vi "Pre-Build Failure Tests.vi"(8 "error in (no error)":errorcluster, 11 "Pre-Build Properties":T1) -> (0 "error out":errorcluster, 3 "Pre-Build Properties dup":T1)   [LabVIEW 2013]
uses:
  pre-build properties -- cluster.ctl
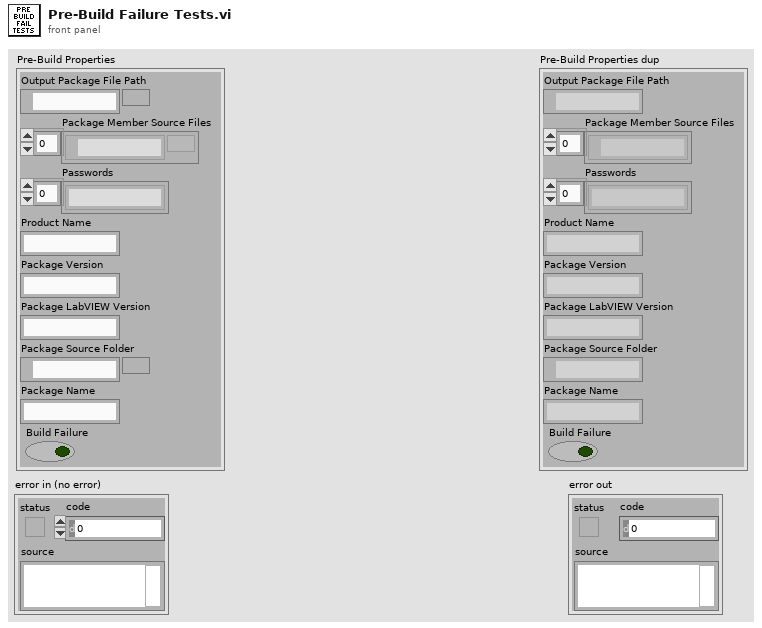
[diagram p1: front panel]
types:
  T1 = typedef "pre-build properties -- cluster.ctl" = cluster{"Output Package File Path":path, "Package Member Source Files":path[], "Passwords":string[], "Product Name":string, "Package Version":string, "Package LabVIEW Version":string, "Package Source Folder":path, "Package Name":string, "Build Failure":bool}
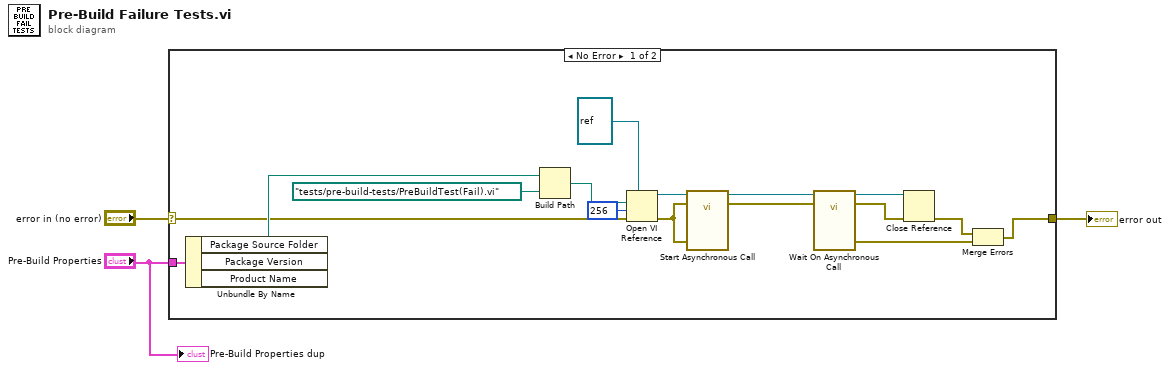
[diagram p0: block diagram]
diagram:
  n1 = case shown="No Error" "error in (no error)" {
    selector: "error in (no error)" -> [w15 w20]
    tunnel: [w9 w20] -> w1
    tunnel: "Pre-Build Properties" -> [w19 _]
    frame No Error {
      n2 = Unbundle By Name(w19) -> ("Package Source Folder"=w18:path)  [unwired: 2 out]
      n3 = Build Path(base path=w18, name or relative path=path "tests/pre-build-tests/PreBuildTest(Fail).vi" ("base path")) -> (appended path=w16:path)
      n4 = Open VI Reference(type specifier VI Refnum (for type only)=refnum<vi> refnum, vi path=w16, options=256, error in (no error)=w15) -> (vi reference=w7:refnum<vi>, error out=w4:errorcluster)  [unwired: 2 in]
      n5 = call-by-ref "Start Asynchronous Call"(reference=w7, error in=w4, 8:"error in (no error)"=w4) -> (reference out=w6:refnum<vi>, error out=w5:errorcluster)  [unwired: 10 in, 1 out]
      n6 = call-by-ref "Wait On Asynchronous Call"(reference=w6, error in=w5) -> (reference out=w13:refnum<vi>, error out=w12:errorcluster, 0:"error out"=w11:errorcluster)  [unwired: 11 in]
      n7 = Close Reference(reference=w13, error in (no error)=w12) -> (error out=w10:errorcluster)
      n8 = Merge Errors(w10, w11) -> (w9:errorcluster)
    }
    frame Error {
    }
  }
  "error out" <- w1
  "Pre-Build Properties dup" <- "Pre-Build Properties"
